vi "example-DeferePanelUpdate.vi"() -> ()   [LabVIEW 2020]
panel:
  in  "Multicolumn Listbox":i32(listbox)
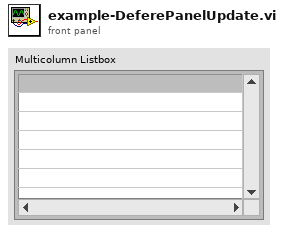
[diagram p1: front panel]
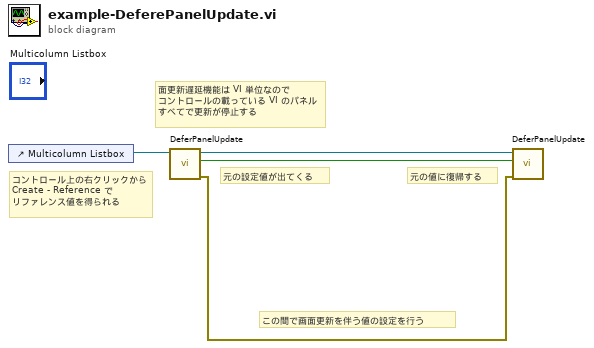
[diagram p0: block diagram]
diagram:
  # "元の設定値が出てくる"
  # "面更新遅延機能は VI 単位なので\nコントロールの載っている VI のパネル\nすべてで更新が停止する"
  # "元の値に復帰する"
  # "この間で画面更新を伴う値の設定を行う"
  # "コントロール上の右クリックから\nCreate - Reference で\nリファレンス値を得られる"
  n1 = control-ref of="Multicolumn Listbox"() -> (w4:refnum<vi>)
  n2 = call "DeferPanelUpdate.vi"("Control in"=w4) -> ("error out"=w1:errorcluster, "Defer Panel Updates Old"=w2:bool, "Control out"=w3:refnum<vi>)  [unwired: 8 in]
  n3 = call "DeferPanelUpdate.vi"("error in (no error)"=w1, "Defer Panel Updates (T)"=w2, "Control in"=w3) -> ()  [unwired: 6 in, 3 out]
